vi "getMeasure.vi"(8 "error in (no error)":errorcluster, 10 "Reading Option (0: Latest)":i32, 11 "Electrometer in":refnum<class "Electrometer.lvclass">) -> (0 "error out":errorcluster, 2 "Measure":dbl, 3 "Electrometer out":refnum<class "Electrometer.lvclass">)   [LabVIEW 2016, in "Electrometer.lvclass"]
uses:
  Electrometer.lvclass
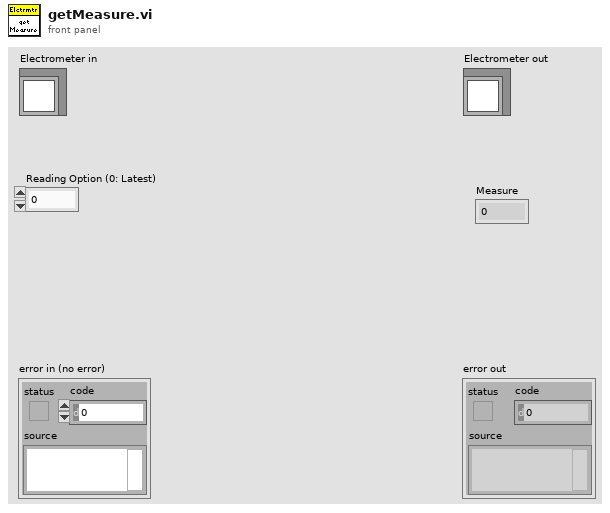
[diagram p1: front panel]
types:
  T1 = cluster{"Measurement":dbl, "Units":string, "Time Stamp and Date":string, "Reading #":dbl, "Channel #":dbl}
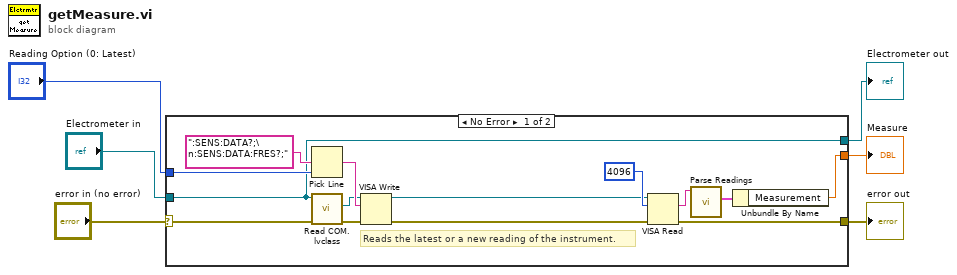
[diagram p0: block diagram]
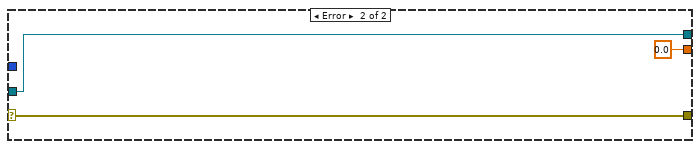
[diagram p2: hidden frame]
diagram:
  n1 = case shown="No Error" "error in (no error)" {
    selector: "error in (no error)" -> [w9 w23]
    tunnel: [w12 w23] -> w5
    tunnel: [w7 w22] -> w3
    tunnel: "Electrometer in" -> [w7 w22]
    tunnel: [w19 0.0 ("Volt 2")] -> w2
    tunnel: "Reading Option (0: Latest)" -> [w11 _]
    frame No Error {
      # "Reads the latest or a new reading of the instrument."
      n2 = Pick Line(multi-line string=":SENS:DATA?;\n:SENS:DATA:FRES?;", line index=w11) -> (output string=w15:string)  [unwired: 1 in]
      n3 = call "Read COM.lvclass.vi"("error in (no error)"=w9, "Electrometer in"=w7) -> ("error out"=w10:errorcluster, "VISA"=w8:refnum<visa-resource-name>)  [unwired: 7 in, 1 out]
      n4 = VISA Write(VISA resource name=w8, write buffer=w15, error in (no error)=w10) -> (VISA resource name out=w17:refnum<visa-resource-name>, error out=w16:errorcluster)  [unwired: 1 out]
      n5 = VISA Read(VISA resource name=w17, byte count=u32 4096, error in (no error)=w16) -> (read buffer=w13:string, error out=w12:errorcluster)  [unwired: 2 out]
      n6 = call "Parse Readings.vi"("Readings"=w13) -> ("Measurement"=w20:T1)  [unwired: 9 in, 1 out]
      n7 = Unbundle By Name(w20) -> ("Measurement"=w19:dbl)
    }
    frame Error {
    }
  }
  "error out" <- w5
  "Electrometer out" <- w3
  "Measure" <- w2
